vi "Database Logging (parameterized).vi"() -> ()   [LabVIEW 2018]
doc: "This example inserts data into a table named logging in the LabVIEW.mdb database. The data is generated and inserted into the database once per second until you press the Stop button. You can use either of the Playback examples to read the data back into LabVIEW.\n\nThis VI uses a parameterized technique to insert data into the database. Since the SQL query can be parsed once and the data is \"filled in\" when needed, this results in a more efficient VI than the Logging Example. However, the parameterized method is more difficult because it requires you to know more about SQL queries and data types."
uses:
  <vilib>/addons/database/Auxilliary.llb/DB Tools Parameter Info.ctl
  <vilib>/addons/database/Auxilliary.llb/DB Tools DataTypes.ctl
  <vilib>/addons/database/Auxilliary.llb/DB Tools Parameter Dir.ctl
  <vilib>/addons/database/Auxilliary.llb/DB Tools Column Info.ctl
  <vilib>/addons/database/Connection.llb/DB Tools Open Connec (Path).vi
  <vilib>/addons/database/Command.llb/Cmd Set Parameter Value (C).vi
  <vilib>/addons/database/Command.llb/Cmd Execute.vi
  <vilib>/addons/database/Recordset.llb/Rec Destroy - Command.vi
  <vilib>/addons/database/Command.llb/Cmd Delete.vi
  <vilib>/addons/database/NI_Database_API.lvlib
panel:
  out "Number of Records":i32=1
  in  "Stop":bool
  out "min temperature value":dbl=296.96037098124657
  out "max temperature value":dbl=403.0350221018737
  out "min pressure value":dbl=0.29112676548258615
  out "max pressure value":dbl=1.56111506192063
  out "Core Temperature":dbl[](graph)
  out "Core Pressure":dbl[](graph)
  # "Overview: Demonstrates the use of a parameterized technique to insert data into a database.\nRequirements: Database Connectivity Toolkit\nInstructions:\n1. Run the VI to log data to the example database.\n2. Open one of the \"Playback\" database examples to display the data that was logged."
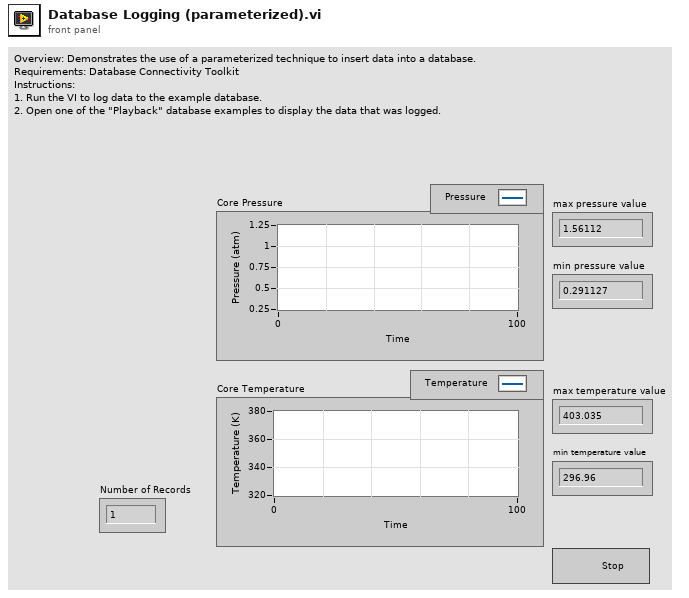
[diagram p1: front panel]
types:
  T1 = typedef "NI_Database_API.lvlib/DB Tools Column Info.ctl" = cluster{"column name":string, "data type":T2, "size":i32, "allow null?":bool}
  T2 = typedef "NI_Database_API.lvlib/DB Tools DataTypes.ctl" = enum16{"String", "Long (I32)", "Single (SGL)", "Double (DBL)", "Date/Time", "Binary"}
  T3 = typedef "NI_Database_API.lvlib/DB Tools Parameter Info.ctl" = cluster{"parameter name":string, "type":T2, "direction":T4, "value":variant}
  T4 = typedef "NI_Database_API.lvlib/DB Tools Parameter Dir.ctl" = enum32{"Input", "Output", "Input/Output", "Return Value"}
  T5 = typedef "NI_Database_API.lvlib/Conn ObjectReference.ctl" = refnum<k1>
  T6 = typedef "NI_Database_API.lvlib/Cmd ObjectReference.ctl" = refnum<k1>
  T7 = typedef "NI_Database_API.lvlib/Cmd-Rec Object Reference.ctl" = refnum<k1>
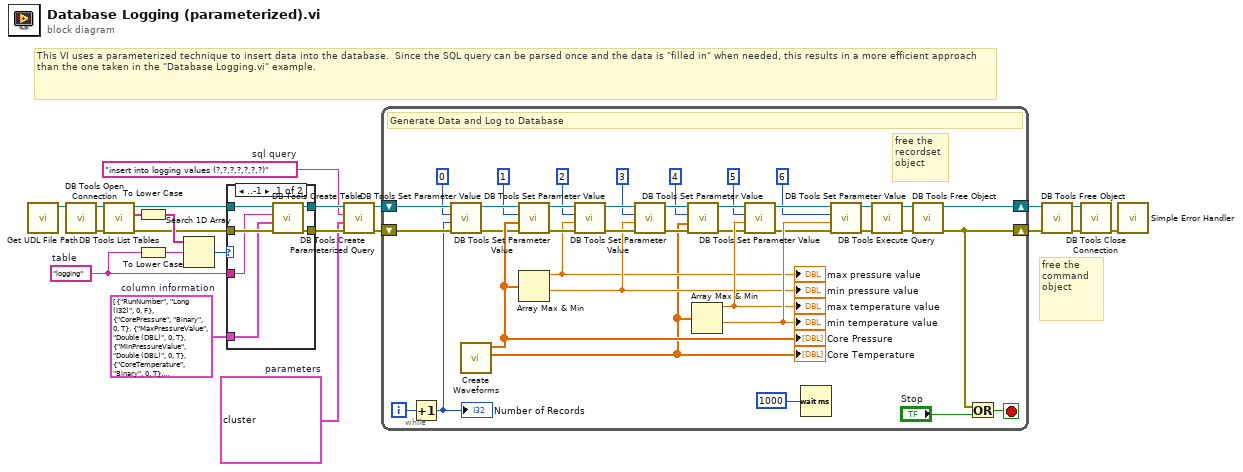
[diagram p0: block diagram]
diagram:
  w6 = T1[] [{"column name"="RunNumber", "data type"=enum."Long (I32)", "size"=0, "allow null?"=FALSE}, {"column name"="CorePressure", "data type"=enum."Binary", "size"=0, "allow null?"=TRUE}, {"column name"="MaxPressureValue", "data type"=enum."Double (DBL)", "size"=0, "allow null?"=TRUE}, {"column name"="MinPressureValue", "data type"=enum."Double (DBL)", "size"=0, "allow null?"=TRUE}, {"column name"="CoreTemperature", "data type"=enum."Binary", "size"=0, "allow null?"=TRUE}, {"column name"="MaxTemperatureValue", "data type"=enum."Double (DBL)", "size"=0, "allow null?"=TRUE}, {"column name"="MinTemperatureValue", "data type"=enum."Double (DBL)", "size"=0, "allow null?"=TRUE}]  # column information
  w19 = T3[] [{"parameter name"="", "type"=enum."Long (I32)", "direction"=enum."Input", "value"=variant}, {"parameter name"="", "type"=enum."Binary", "direction"=enum."Input", "value"=variant}, {"parameter name"="", "type"=enum."Double (DBL)", "direction"=enum."Input", "value"=variant}, {"parameter name"="", "type"=enum."Double (DBL)", "direction"=enum."Input", "value"=variant}, {"parameter name"="", "type"=enum."Binary", "direction"=enum."Input", "value"=variant}, {"parameter name"="", "type"=enum."Double (DBL)", "direction"=enum."Input", "value"=variant}, {"parameter name"="", "type"=enum."Double (DBL)", "direction"=enum."Input", "value"=variant}]  # parameters
  w20 = "insert into logging values (?,?,?,?,?,?,?)"  # sql query
  w9 = "logging"  # table
  # "free the command object"
  # "This VI uses a parameterized technique to insert data into the database.  Since the SQL query can be parsed once and the data is \"filled in\" when needed, this results in a more efficient approach than the one taken in the \"Database Logging.vi\" example."
  n1 = call "Get UDL File Path.vi"() -> ("UDL file path"=w5:path)  [unwired: 11 in]
  n2 = call-poly <vilib>:"DB Tools Open Connection.vi"("connection information"=w5) -> ("error out"=w13:errorcluster, "connection reference"=w12:T5)  [unwired: 7 in]
  n3 = call <vilib>:"DB Tools List Tables.vi"("error in (no error)"=w13, "connection reference"=w12) -> ("error out"=w8:errorcluster, "tables"=w10:string[], "connection reference out"=w7:T5)  [unwired: 3 in]
  n4 = To Lower Case(string=w10) -> (all lower case string=w11:string[])
  n5 = To Lower Case(string=w9) -> (all lower case string=w2:string)
  n6 = Search 1D Array(1D array=w11, element=w2) -> (index of element=w3:i32)  [unwired: 1 in]
  n7 = case shown="..-1" w3 {
    tunnel: w7 -> [w27 w30]
    tunnel: w8 -> [w28 w29]
    tunnel: [w26 w30] -> w21
    tunnel: [w25 w29] -> w22
    tunnel: w9 -> [w24 _]
    tunnel: w6 -> [w23 _]
    frame ..-1 {
      n8 = call <vilib>:"DB Tools Create Table.vi"("error in (no error)"=w28, "column information"=w23, "table"=w24, "connection reference"=w27) -> ("error out"=w25:errorcluster, "connection reference out"=w26:T5)  [unwired: 4 in]
    }
    frame 0.. {
    }
  }
  n9 = call <vilib>:"DB Tools Create Parameterized Query.vi"("error in (no error)"=w22, "parameters"=w19, "SQL query"=w20, "connection reference"=w21) -> ("error out"=w15:errorcluster, "command reference"=w18:T6)  [unwired: 3 in, 1 out]
  n10 = while {
    shift-right: [w40] -> w17
    shift-left: w15 -> [w47]
    shift-right: [w31] -> w1
    shift-left: w18 -> [w48]
    i -> [w66]
    stop <- w64 stop-if-true
    # "free the recordset object"
    # "Generate Data and Log to Database"
    n11 = Increment(x=w66) -> (x+1=w44:i32)
    "Number of Records" <- w44
    n12 = call-poly <vilib>:"DB Tools Set Parameter Value.vi"("error in (no error)"=w47, "value"=w44, "parameter index"=0, "command reference"=w48) -> ("error out"=w46:errorcluster, "command reference out"=w45:T6)  [unwired: 4 in]
    n13 = call "Create Waveforms.vi"() -> ("core temperature"=w41:dbl[], "core pressure"=w51:dbl[])  [unwired: 10 in]
    "Core Pressure" <- w51
    "Core Temperature" <- w41
    n14 = call-poly <vilib>:"DB Tools Set Parameter Value.vi"("error in (no error)"=w46, "value"=w51, "parameter index"=1, "command reference"=w45) -> ("error out"=w63:errorcluster, "command reference out"=w62:T6)  [unwired: 4 in]
    n15 = Array Max & Min(array=w51) -> (max value=w50:dbl, min value=w53:dbl)  [unwired: 2 out]
    "max pressure value" <- w50
    "min pressure value" <- w53
    n16 = call-poly <vilib>:"DB Tools Set Parameter Value.vi"("error in (no error)"=w63, "value"=w50, "parameter index"=2, "command reference"=w62) -> ("error out"=w61:errorcluster, "command reference out"=w49:T6)  [unwired: 4 in]
    n17 = call-poly <vilib>:"DB Tools Set Parameter Value.vi"("error in (no error)"=w61, "value"=w53, "parameter index"=3, "command reference"=w49) -> ("error out"=w60:errorcluster, "command reference out"=w43:T6)  [unwired: 4 in]
    n18 = call-poly <vilib>:"DB Tools Set Parameter Value.vi"("error in (no error)"=w60, "value"=w41, "parameter index"=4, "command reference"=w43) -> ("error out"=w59:errorcluster, "command reference out"=w58:T6)  [unwired: 4 in]
    n19 = Array Max & Min(array=w41) -> (max value=w67:dbl, min value=w68:dbl)  [unwired: 2 out]
    "max temperature value" <- w67
    "min temperature value" <- w68
    n20 = call-poly <vilib>:"DB Tools Set Parameter Value.vi"("error in (no error)"=w59, "value"=w67, "parameter index"=5, "command reference"=w58) -> ("error out"=w56:errorcluster, "command reference out"=w57:T6)  [unwired: 4 in]
    n21 = Wait (ms)(milliseconds to wait=u32 1000) -> ()  [unwired: 1 out]
    n22 = call-poly <vilib>:"DB Tools Set Parameter Value.vi"("error in (no error)"=w56, "value"=w68, "parameter index"=6, "command reference"=w57) -> ("error out"=w42:errorcluster, "command reference out"=w52:T6)  [unwired: 4 in]
    n23 = call-poly <vilib>:"DB Tools Execute Query.vi"("error in (no error)"=w42, "command reference"=w52) -> ("error out"=w55:errorcluster, "command-recordset reference"=w54:T7)  [unwired: 6 in]
    n24 = call-poly <vilib>:"DB Tools Free Object.vi"("error in (no error)"=w55, "command-recordset reference"=w54) -> ("error out"=w40:errorcluster, "command reference"=w31:T6)  [unwired: 8 in]
    n25 = Or(x=w40, y="Stop") -> (x .or. y?=w64:bool)
  }
  n26 = call-poly <vilib>:"DB Tools Free Object.vi"("error in (no error)"=w17, "command reference"=w1) -> ("error out"=w16:errorcluster, "connection reference"=w4:T5)  [unwired: 8 in]
  n27 = call <vilib>:"DB Tools Close Connection.vi"("error in (no error)"=w16, "connection reference"=w4) -> ("error out"=w14:errorcluster)  [unwired: 5 in]
  n28 = call <vilib>:"Simple Error Handler.vi"("error in (no error)"=w14) -> ()  [unwired: 4 in, 5 out]
